vi "read.vi"(7 "timeout (ms)":i32, 8 "error in (no error)":errorcluster, 9 "number of channels":i32, 10 "block size":i32, 11 "FPGAWrapperDL090211Galvo in":refnum<class "FPGAWrapperDL090211Galvo.lvclass">) -> (0 "error out":errorcluster, 1 "channels raw data block":T1, 2 "FIFO full?":bool, 3 "FPGAWrapperDL090211Galvo out":refnum<class "FPGAWrapperDL090211Galvo.lvclass">, 4 "timed out?":bool)   [LabVIEW 2010, in "FPGAWrapperDL090211Galvo.lvclass"]
uses:
  FPGAWrapperDL090211Galvo.lvclass
  common/arrays/pixel_raw_data_array.ctl
  GenericFPGAWrapper/GenericFPGAWrapper/GenericFPGAWrapper.lvclass
  <vilib>/rvi/interface/nirviReadWriteControl/nirviReadWriteControl.xnode
  FPGA_VI_ref.ctl
  <vilib>/rvi/interface/common/niFpgaNodeNameForErrorReporting.ctl
  <vilib>/rvi/errors/niLvFpgaWhatHappensToTopLevelVI.ctl
  <vilib>/rvi/interface/nirviMethod/nirviMethod.xnode
  <vilib>/Utility/error.llb/Error Cluster From Error Code.vi
  <vilib>/rvi/errors/niLvFpgaAdjustHostInterfaceError.vi
  NiFpgaLv.dll
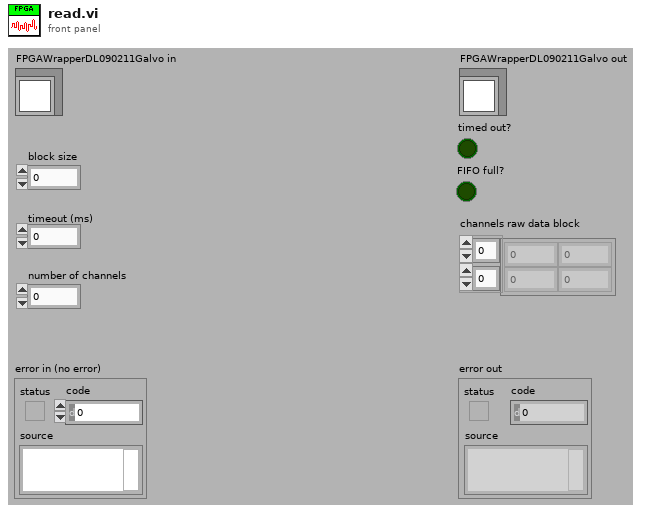
[diagram p1: front panel]
types:
  T1 = typedef "pixel_raw_data_array.ctl" = dbl[][]
  T2 = typedef "niFpgaNodeNameForErrorReporting.ctl" = enum16{"Open FPGA VI Reference", "Read/Write Control", "Invoke Method: Abort", "Invoke Method: Acknowledge IRQ", "Invoke Method: Download", "Invoke Method: FIFO.Configure", "Invoke Method: FIFO.Read", "Invoke Method: FIFO.Start", "Invoke Method: FIFO.Stop", "Invoke Method: FIFO.Write", "Invoke Method: Reset", "Invoke Method: Run", "Invoke Method: Wait on IRQ", "Close FPGA VI Reference"}
  T3 = typedef "niLvFpgaWhatHappensToTopLevelVI.ctl" = enum16{"top level VI scripted behind XNode", "top level VI inlined behind XNode"}
  T4 = typedef "FPGAWrapperDL090211Galvo.lvclass/FPGA_VI_ref.ctl" = refnum<k20>
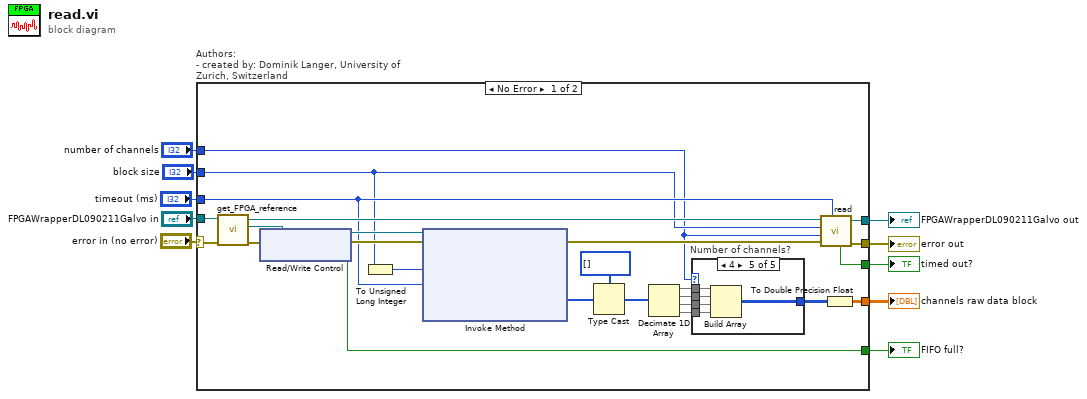
[diagram p0: block diagram]
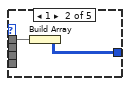
[diagram p3: hidden frame]
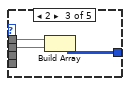
[diagram p4: hidden frame]
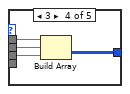
[diagram p5: hidden frame]
diagram:
  n1 = case "Authors: \n- created by: Dominik Langer, University of Zurich, Switzerland" shown="No Error" "error in (no error)" {
    selector: "error in (no error)" -> [w35 w166]
    tunnel: "FPGAWrapperDL090211Galvo in" -> [w28 w167]
    tunnel: "timeout (ms)" -> [w25 _]
    tunnel: "number of channels" -> [w14 _]
    tunnel: "block size" -> [w16 _]
    tunnel: [w30 _] -> w5
    tunnel: [w24 w166] -> w4
    tunnel: [w23 w167] -> w3
    tunnel: [w29 _] -> w2
    tunnel: [w17 _] -> w1
    frame No Error {
      n2 = call-dynamic "get_FPGA_reference.vi"("error in (no error)"=w35, "FPGAWrapperDL090211Galvo in"=w28) -> ("error out"=w34:errorcluster, "FPGA VI reference"=w33:T4, "FPGAWrapperDL090211Galvo out"=w31:refnum<class "FPGAWrapperDL090211Galvo.lvclass">)  [unwired: 6 in, 1 out]
      n3 = xnode "Read/Write Control"("FPGA VI Reference In"=w33, "error in"=w34) -> ("FPGA VI Reference Out"=w26:T4, "error out"=w32:errorcluster, "FIFO overflow"=w29:bool)
      n4 = To Unsigned Long Integer(number=w16) -> (unsigned 32bit integer=w15:u32)
      n5 = xnode "Invoke Method"("FPGA VI Reference In"=w26, "error in"=w32, "Number of Elements"=w15, "Timeout (ms)"=w25) -> ("error out"=w27:errorcluster, "Data"=w13:u64[])  [unwired: 2 out]
      n6 = Type Cast(type=u16[] [], x=w13) -> (*(type *) &x=w12:u16[])
      n7 = Decimate 1D Array(w12) -> (w22:u16[], w21:u16[], w20:u16[], w19:u16[])
      n8 = case "Number of channels?" shown="4" w14 {
        tunnel: w22 -> [_ w37 w40 w44 w49]
        tunnel: w21 -> [_ _ w39 w43 w48]
        tunnel: w20 -> [_ _ _ w42 w47]
        tunnel: w19 -> [_ _ _ _ w46]
        tunnel: [_ w36 w38 w41 w45] -> w18
        frame 0, Default {
        }
        frame 1 {
          n9 = Build Array(w37) -> (w36:u16[][])
        }
        frame 2 {
          n10 = Build Array(w40, w39) -> (w38:u16[][])
        }
        frame 3 {
          n11 = Build Array(w44, w43, w42) -> (w41:u16[][])
        }
        frame 4 {
          n12 = Build Array(w49, w48, w47, w46) -> (w45:u16[][])
        }
      }
      n13 = call-parent "read.vi"("timeout (ms)"=w25, "error in (no error)"=w27, "number of channels"=w14, "block size"=w16, "GenericFPGAWrapper in"=w31) -> ("error out"=w24:errorcluster, "GenericFPGAWrapper out"=w23:refnum<class "FPGAWrapperDL090211Galvo.lvclass">, "timed out?"=w30:bool)  [unwired: 2 in, 2 out]
      n14 = To Double Precision Float(number=w18) -> (double precision float=w17:dbl[][])
    }
    frame Error {
    }
  }
  "error out" <- w4
  "FPGAWrapperDL090211Galvo out" <- w3
  "FIFO full?" <- w2
  "channels raw data block" <- w1
  "timed out?" <- w5
